vi "Stop Core.vi"(10 "final error code":i32, 11 "Client Controller in":refnum<class "Client Controller.lvclass">) -> (3 "Client Controller out":refnum<class "Client Controller.lvclass">)   [LabVIEW 2015, in "Client Controller.lvlib" / "Client Controller.lvclass"]
uses:
  Client Controller.lvclass
  Client Controller.lvclass/Client Controller.ctl
  <vilib>/ActorFramework/Message Enqueuer/Message Enqueuer.lvclass/Message Enqueuer.ctl
  <vilib>/ActorFramework/Message Enqueuer/Enqueue.vi
  <vilib>/ActorFramework/Message Priority Queue/Priority Enqueue.vi
  <vilib>/ActorFramework/Message Enqueuer/Message Enqueuer.lvclass
  <vilib>/ActorFramework/Stop Msg/Stop Msg.lvclass
  <userlib>/Configuration Dialog Actor/Configuration.lvclass
  <userlib>/Common Components/Controller/Controller.lvclass
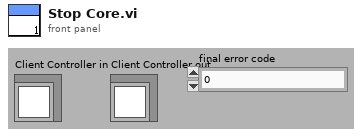
[diagram p1: front panel]
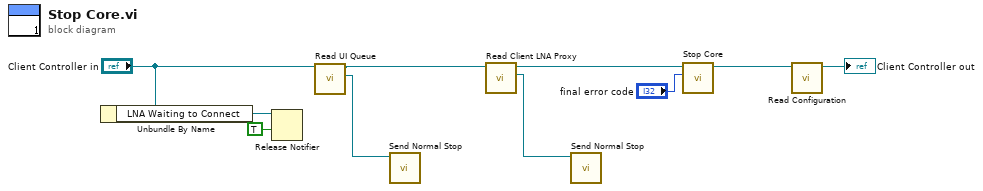
[diagram p0: block diagram]
diagram:
  n1 = Unbundle By Name("Client Controller in") -> ("LNA Waiting to Connect"=w4:refnum<notifier>)
  n2 = Release Notifier(notifier=w4, force destroy? (F)=TRUE) -> ()  [unwired: 1 in, 3 out]
  n3 = call <userlib>:"Read UI Queue.vi"("UI Controller in"="Client Controller in") -> ("UI Queue"=w7:refnum<class "Message Enqueuer.lvclass">, "UI Controller out"=w8:refnum<class "Client Controller.lvclass">)  [unwired: 8 in, 1 out]
  n4 = call <vilib>:"Send Normal Stop.vi"("Message Enqueuer"=w7) -> ()  [unwired: 10 in, 1 out]
  n5 = call "Read Client LNA Proxy.vi"("Client Controller in"=w8) -> ("Actor Framework:Message Enqueuer"=w9:refnum<class "Message Enqueuer.lvclass">, "Client Controller out"=w6:refnum<class "Client Controller.lvclass">)  [unwired: 8 in, 1 out]
  n6 = call <vilib>:"Send Normal Stop.vi"("Message Enqueuer"=w9) -> ()  [unwired: 10 in, 1 out]
  n7 = call-parent "Stop Core.vi"("final error code"="final error code", "Controller in"=w6) -> ("Controller out"=w2:refnum<class "Client Controller.lvclass">)  [unwired: 9 in]
  n8 = call <userlib>:"Read Configuration.vi"("Controller in"=w2) -> ("Controller out"=→"Client Controller out":refnum<class "Client Controller.lvclass">)  [unwired: 8 in, 2 out]
